vi "Convert Data For Intensity Graph.vi"(9 "Reader index":i32, 10 "Data In":cluster{cluster{"x":T1, "x":T1}[]}[](array[cluster])) -> (0 "min value":T1, 1 "max value":T1, 2 "Data out":T1[][](array[typedef]), 3 "bounds":cluster{T1, T1, T1, T1})   [LabVIEW 2015, in "Scan Driver.lvclass"]
uses:
  Scan Driver.lvclass
  Instruments/Utility Classes/Readable/X.ctl
  Instruments/Utility Classes/Readable/Readable.lvclass
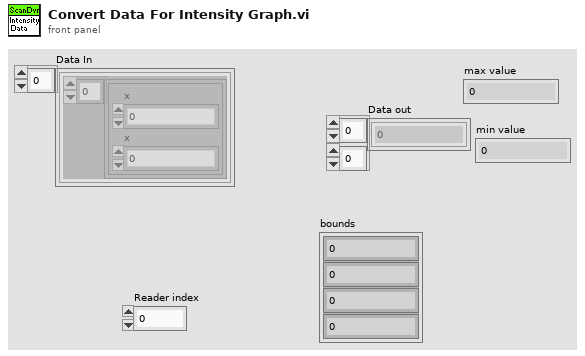
[diagram p1: front panel]
types:
  T1 = typedef "Readable.lvclass/X.ctl" = dbl
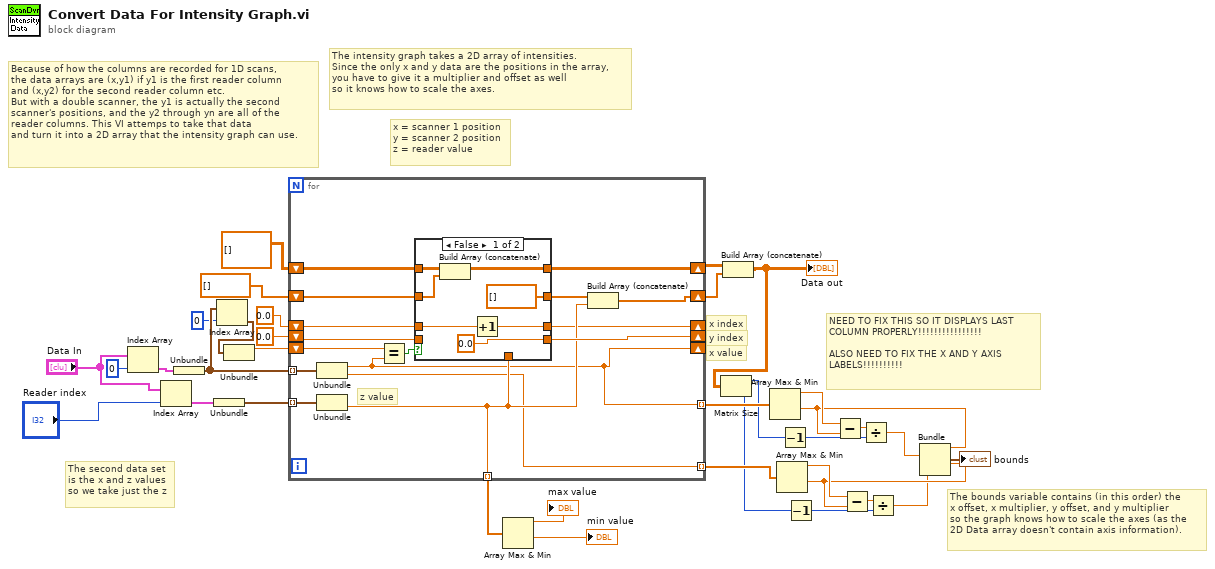
[diagram p0: block diagram]
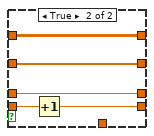
[diagram p2: hidden frame]
diagram:
  # "The bounds variable contains (in this order) the\nx offset, x multiplier, y offset, and y multiplier \nso the graph knows how to scale the axes (as the\n2D Data array doesn't contain axis information)."
  # "NEED TO FIX THIS SO IT DISPLAYS LAST\nCOLUMN PROPERLY!!!!!!!!!!!!!!!!\n\nALSO NEED TO FIX THE X AND Y AXIS\nLABELS!!!!!!!!!!"
  # "x = scanner 1 position\ny = scanner 2 position\nz = reader value"
  # "x value"
  # "y index"
  # "x index"
  # "The second data set\nis the x and z values\nso we take just the z"
  # "Because of how the columns are recorded for 1D scans, \nthe data arrays are (x,y1) if y1 is the first reader column \nand (x,y2) for the second reader column etc. \nBut with a double scanner, the y1 is actually the second \nscanner's positions, and the y2 through yn are all of the\nreader columns. This VI attemps to take that data\nand turn it into a 2D array that the intensity graph can use."
  # "The intensity graph takes a 2D array of intensities. \nSince the only x and y data are the positions in the array, \nyou have to give it a multiplier and offset as well \nso it knows how to scale the axes."
  n1 = Index Array(array="Data In", index=0) -> (element=w34:cluster{cluster{"x":T1, "x":T1}[]})
  n2 = Index Array(array="Data In", index="Reader index") -> (element=w33:cluster{cluster{"x":T1, "x":T1}[]})
  n3 = Unbundle(w34) -> (w28:cluster{"x":T1, "x":T1}[])
  n4 = Unbundle(w33) -> (w31:cluster{"x":T1, "x":T1}[])
  n5 = Index Array(array=w28, index=0) -> (element=w26:cluster{"x":T1, "x":T1})
  n6 = Unbundle(w26) -> ("x"=w25:T1)  [unwired: 1 out]
  n7 = for {
    tunnel: w28 -> [w51] mode=indexing
    tunnel: w31 -> [w50] mode=indexing
    shift-right: [w37] -> _
    shift-left: w25 -> [w48]
    shift-right: [w38] -> _
    shift-left: 0.0 -> [w47]
    shift-right: [w42] -> _
    shift-left: 0.0 -> [w46]
    shift-right: [w43] -> w4
    shift-left: T1[][] [] ("Data out") -> [w44]
    tunnel: [w39] -> w22 mode=indexing
    shift-right: [w40] -> w3
    shift-left: dbl[] [] ("array") -> [w45]
    tunnel: [w37] -> w18 mode=indexing
    tunnel: [w36] -> w12 mode=indexing
    # "z value"
    n8 = Unbundle(w51) -> ("x"=w37:T1, "x"=w36:T1)
    n9 = Unbundle(w50) -> ("x"=w39:T1)  [unwired: 1 out]
    n10 = Equal?(x=w48, y=w37) -> (x = y?=w49:bool)
    n11 = case shown="False" w49 {
      tunnel: [w58 w63] -> w38
      tunnel: w47 -> [w54 w63]
      tunnel: [0.0 w62] -> w42
      tunnel: w46 -> [_ w61]
      tunnel: w39 -> [_ _]
      tunnel: w45 -> [w52 w60]
      tunnel: w44 -> [w55 w59]
      tunnel: [w53 w59] -> w43
      tunnel: [dbl[] [] ("array") w60] -> w41
      frame False {
        n12 = Build Array (concatenate)(w55, w52) -> (w53:T1[][])
        n13 = Increment(x=w54) -> (x+1=w58:dbl)
      }
      frame True {
        n14 = Increment(x=w61) -> (x+1=w62:dbl)
      }
    }
    n15 = Build Array (concatenate)(w41, w39) -> (w40:T1[])
  }
  n16 = Array Max & Min(array=w22) -> (max value=→"max value":T1, min value=→"min value":T1)  [unwired: 2 out]
  n17 = Build Array (concatenate)(w4, w3) -> (w2:T1[][])
  "Data out" <- w2
  n18 = Matrix Size(0:w2) -> (1:w6:i32, 2:w5:i32)
  n19 = Array Max & Min(array=w18) -> (max value=w19:T1, min value=w11:T1)  [unwired: 2 out]
  n20 = Array Max & Min(array=w12) -> (max value=w15:T1, min value=w9:T1)  [unwired: 2 out]
  n21 = Decrement(x=w6) -> (x-1=w16:i32)
  n22 = Decrement(x=w5) -> (x-1=w13:i32)
  n23 = Subtract(x=w19, y=w11) -> (x-y=w17:T1)
  n24 = Subtract(x=w15, y=w9) -> (x-y=w14:T1)
  n25 = Divide(x=w17, y=w16) -> (x/y=w10:T1)
  n26 = Divide(x=w14, y=w13) -> (x/y=w8:T1)
  n27 = Bundle(w11, w10, w9, w8) -> (→"bounds":cluster{T1, T1, T1, T1})  [unwired: 1 in]
